vi "Get All Users.vi"(0 "User Configuration Manager in":refnum<class "User Configuration Manager.lvclass">, 11 "error in (no error)":errorcluster) -> (4 "User Configuration Manager out":refnum<class "User Configuration Manager.lvclass">, 6 "Users":string[](array[string]), 8 "Number of Users Found":u32, 15 "error out":errorcluster)   [LabVIEW 2019, in "User Configuration Manager.lvlib" / "User Configuration Manager.lvclass"]
uses:
  <vilib>/gpm_packages/@cs/user-manager/Source/User Configuration Manager/User Configuration Manager.lvclass
  <vilib>/gpm_packages/@cs/user-manager/Source/User Configuration Manager/User Configuration Manager.lvclass/User Configuration Manager.ctl
  <vilib>/gpm_packages/@cs/user-manager/Source/User Configuration Manager/Accessors/Read Linked List ID.vi
  <vilib>/gpm_packages/@cs/user-manager/Source/User Configuration Manager/Accessors/Read Linked List Ref .vi
  <vilib>/gpm_packages/@cs/linked-list/Source/Linked List/ILinkedList/ILinked List.lvclass
  <vilib>/gpm_packages/@cs/linked-list/Source/Linked List/Linked List Ref/Linked List Ref.lvclass
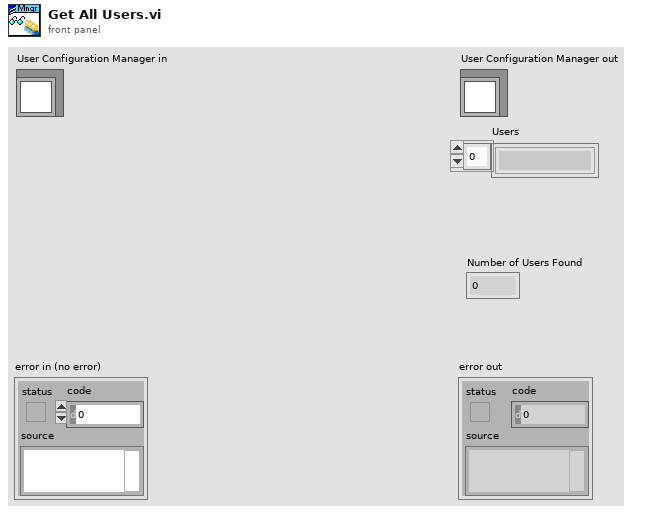
[diagram p1: front panel]
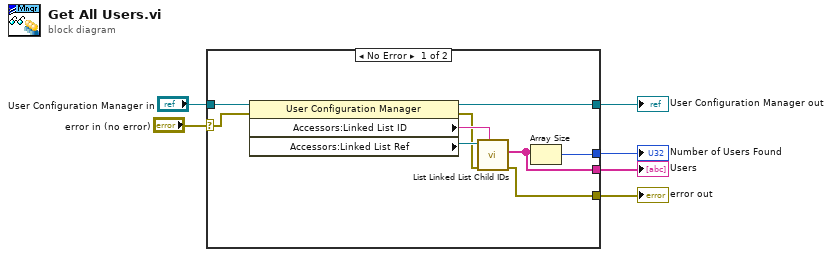
[diagram p0: block diagram]
diagram:
  n1 = case shown="No Error" "error in (no error)" {
    selector: "error in (no error)" -> [w13 w17]
    tunnel: "User Configuration Manager in" -> [w15 w16]
    tunnel: [w14 w16] -> w5
    tunnel: [w9 _] -> w3
    tunnel: [w7 w17] -> w2
    tunnel: [w10 _] -> w1
    frame No Error {
      n2 = property class="User Configuration Manager"(reference=w15, error in=w13) -> (reference out=w14:refnum<class "User Configuration Manager.lvclass">, error out=w8:errorcluster, "Accessors:Linked List ID"=w11:string, "Accessors:Linked List Ref "=w12:refnum<data-value>)
      n3 = call <vilib>:"List Linked List Child IDs.vi"("Linked List ID"=w11, "error in (no error)"=w8, "Linked List Ref"=w12) -> ("error out"=w7:errorcluster, "Child IDs"=w10:string[])  [unwired: 6 in, 1 out]
      n4 = Array Size(array=w10) -> (size(s)=w9:i32)
    }
    frame Error {
    }
  }
  "error out" <- w2
  "User Configuration Manager out" <- w5
  "Users" <- w1
  "Number of Users Found" <- w3
